vi "_Read_D.vi"(8 "error in (no error)":errorcluster, 11 "Postgres Connector In":refnum<class "Postgres Connector.lvclass">) -> (0 "error out":errorcluster, 3 "Postgres Connector Out":refnum<class "Postgres Connector.lvclass">)   [LabVIEW 2019, in "PG_LIB.lvlib" / "Postgres Connector.lvclass"]
doc: "This VI decode the \"D\" section of the message sent by the database and return the value of each rows."
uses:
  Postgres Connector.lvclass
  Enum_RowDescription_State_Machine.ctl
  Cluster_Reader_Infos.ctl
  Postgres Connector.lvclass/Postgres Connector.ctl
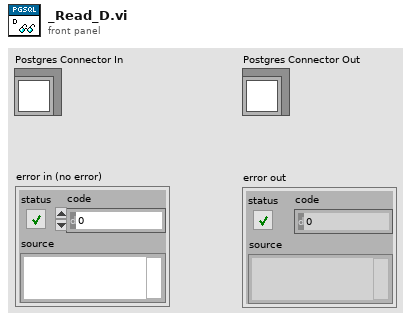
[diagram p1: front panel]
types:
  T1 = typedef "PG_LIB.lvlib/Postgres Connector.lvclass/Cluster_Reader_Infos.ctl" = cluster{"Byte Length":i32}
  T2 = typedef "PG_LIB.lvlib/Postgres Connector.lvclass/Enum_RowDescription_State_Machine.ctl" = enum16{"Check For Error", "Wait For T", "Wait For D", "Wait For Z", "C Byte Length", "Z Byte Length", "n Byte Length", "Byte Length", "Get Infos", "Check For End", "Flush", "Quit"}
  T3 = enum16{"Standard", "Buffered", "CRLF", "Immediate"}
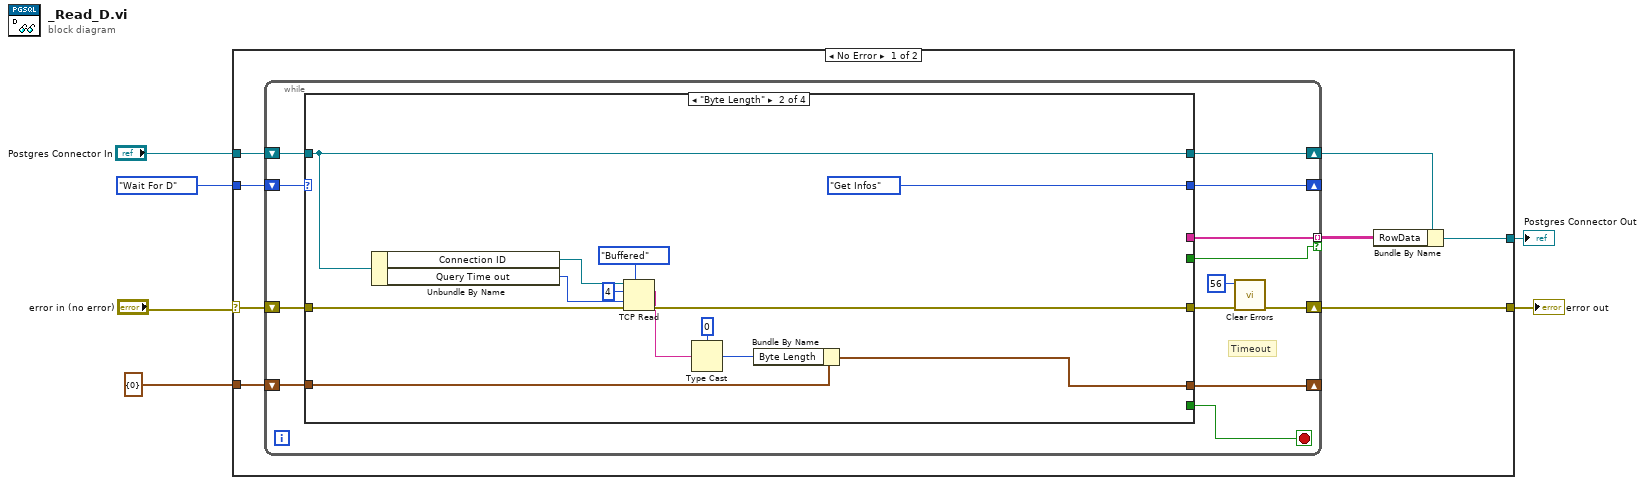
[diagram p0: block diagram]
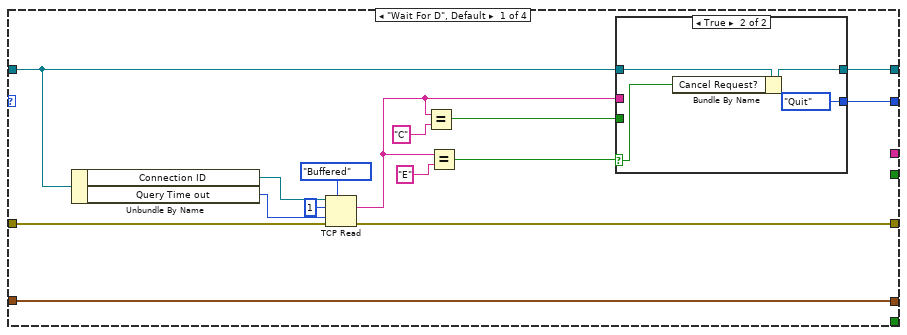
[diagram p2: hidden frame]
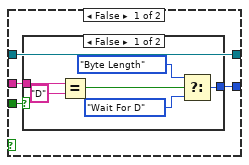
[diagram p3: hidden frame]
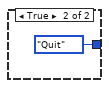
[diagram p4: hidden frame]
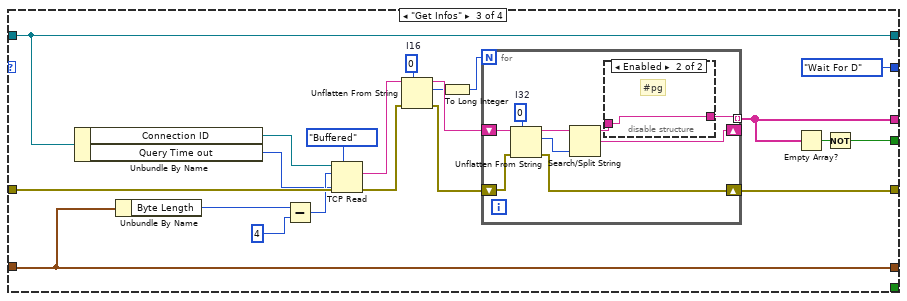
[diagram p5: hidden frame]
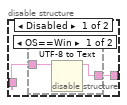
[diagram p6: hidden frame]
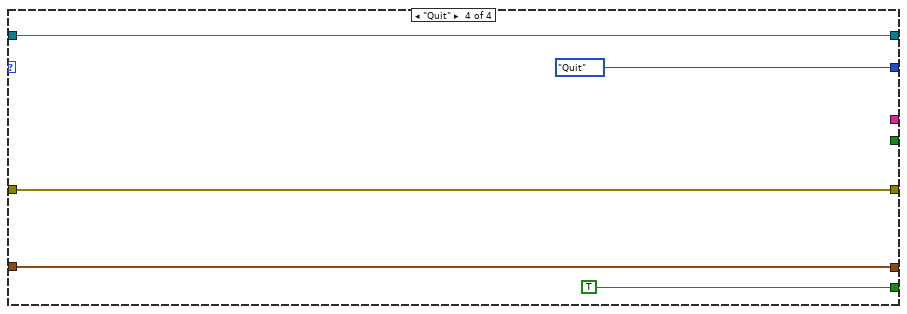
[diagram p8: hidden frame]
diagram:
  n1 = case shown="No Error" "error in (no error)" {
    selector: "error in (no error)" -> [w14 w113]
    tunnel: "Postgres Connector In" -> [w10 w112]
    tunnel: Enum_RowDescription_State_Machine."Wait For D" -> [w13 _]
    tunnel: [w12 w113] -> w3
    tunnel: T1 {"Byte Length"=0} ("Reader_Infos") -> [w11 _]
    tunnel: [w8 w112] -> w1
    frame No Error {
      n2 = while {
        shift-right: [w23] -> w12
        shift-left: w14 -> [w26]
        shift-right: [w21] -> _
        shift-left: w13 -> [w25]
        shift-right: [w19] -> _
        shift-left: w11 -> [w20]
        tunnel: [w17] -> w9 mode=indexing if=w16
        shift-right: [w15] -> w7
        shift-left: w10 -> [w27]
        stop <- w18 stop-if-true
        # "Timeout"
        n3 = case shown="\"Byte Length\"" w25 {
          tunnel: w27 -> [w29 w67 w83 w107]
          tunnel: w26 -> [w39 w66 w89 w110]
          tunnel: [w38 w65 w73 w110] -> w24
          tunnel: [w37 Enum_RowDescription_State_Machine."Get Infos" Enum_RowDescription_State_Machine."Wait For D" Enum_RowDescription_State_Machine."Quit"] -> w21
          tunnel: w20 -> [w36 w63 w87 w111]
          tunnel: [w36 w62 w87 w111] -> w19
          tunnel: [_ _ _ TRUE] -> w18
          tunnel: [_ _ w77 _] -> w17
          tunnel: [_ _ w81 _] -> w16
          tunnel: [w28 w67 w83 w107] -> w15
          frame "Wait For D", Default {
            n4 = Unbundle By Name(w29) -> ("Connection ID"=w41:refnum<k5>, "Query Time out"=w33:i32)
            n5 = TCP Read(connection ID=w41, bytes to read=1, error in (no error)=w39, 7:T3."Buffered" ("mode (standard)"), 9:w33) -> (data out=w31:string, error out=w38:errorcluster)  [unwired: 1 out]
            n6 = Equal?(x=w31, y="C") -> (x = y?=w34:bool)
            n7 = Equal?(x=w31, y="E") -> (x = y?=w30:bool)
            n8 = case shown="True" w30 {
              selector: w30 -> [_ w55]
              tunnel: [w46 Enum_RowDescription_State_Machine."Quit"] -> w37
              tunnel: w34 -> [w45 _]
              tunnel: w31 -> [w44 _]
              tunnel: w29 -> [w43 w56]
              tunnel: [w43 w54] -> w28
              frame False {
                n9 = case shown="False" w45 {
                  tunnel: [w50 Enum_RowDescription_State_Machine."Quit"] -> w46
                  tunnel: w44 -> [w47 _]
                  frame False {
                    n10 = Equal?(x=w47, y="D") -> (x = y?=w51:bool)
                    n11 = Select(t=Enum_RowDescription_State_Machine."Byte Length", s=w51, f=Enum_RowDescription_State_Machine."Wait For D") -> (s? t:f=w50:T2)
                  }
                  frame True {
                  }
                }
              }
              frame True {
                n12 = Bundle By Name(cluster=w56, "Cancel Request?"=w55) -> (w54:refnum<class "Postgres Connector.lvclass">)
              }
            }
          }
          frame "Byte Length" {
            n13 = Unbundle By Name(w67) -> ("Connection ID"=w69:refnum<k5>, "Query Time out"=w58:i32)
            n14 = TCP Read(connection ID=w69, bytes to read=4, error in (no error)=w66, 7:T3."Buffered" ("mode (standard)"), 9:w58) -> (data out=w60:string, error out=w65:errorcluster)  [unwired: 1 out]
            n15 = Type Cast(type=0, x=w60) -> (*(type *) &x=w59:i32)
            n16 = Bundle By Name(cluster=w63, "Byte Length"=w59) -> (w62:T1)
          }
          frame "Get Infos" {
            w80 = i16 0  # I16
            n17 = Unbundle By Name(w83) -> ("Connection ID"=w90:refnum<k5>, "Query Time out"=w74:i32)
            n18 = Unbundle By Name(w87) -> ("Byte Length"=w86:i32)
            n19 = Subtract(x=w86, y=4 ("bytes to read")) -> (x-y=w85:i32)
            n20 = TCP Read(connection ID=w90, bytes to read=w85, error in (no error)=w89, 7:T3."Buffered" ("mode (standard)"), 9:w74) -> (data out=w79:string, error out=w72:errorcluster)  [unwired: 1 out]
            n21 = Unflatten From String(type=w80, binary string=w79, error in (no error)=w72) -> (rest of the binary string=w78:string, value=w76:i16, error out=w71:errorcluster)  [unwired: 2 in]
            n22 = To Long Integer(number=w76) -> (32bit integer=w75:i32)
            n23 = for {
              N: w75 -> [_]
              tunnel: [w92] -> w77 mode=indexing
              shift-right: [w96] -> _
              shift-left: w78 -> [w99]
              shift-right: [w94] -> w73
              shift-left: w71 -> [w95]
              w100 = 0  # I32
              n24 = Unflatten From String(type=w100, binary string=w99, error in (no error)=w95) -> (rest of the binary string=w97:string, value=w98:i32, error out=w94:errorcluster)  [unwired: 2 in]
              n25 = Search/Split String(string=w97, offset (0)=w98) -> (substring before match=w93:string, match + rest of string=w96:string)  [unwired: 1 in, 1 out]
              n26 = disable-structure shown="Enabled" {
                disable-tunnel: w93 -> [w102 w106]
                disable-tunnel: [w101 w106] -> w92
                frame Disabled {
                  n27 = disable-structure shown="OS==Win" {
                    disable-tunnel: w102 -> [w104 w105]
                    disable-tunnel: [w103 w105] -> w101
                    frame condition #0 {
                      n28 = UTF-8 to Text(11:w104) -> (3:w103:string)  [unwired: 2 in, 1 out]
                    }
                    frame condition #1 (active) {
                    }
                  }
                }
                frame Enabled {
                  # "#pg"
                }
              }
            }
            n29 = Empty Array?(array=w77) -> (empty?=w82:bool)
            n30 = Not(x=w82) -> (.not. x?=w81:bool)
          }
          frame "Quit" {
          }
        }
        n31 = call <vilib>:"Clear Errors.vi"("error in (no error)"=w24, "specific error code to clear (0: all)"=56) -> ("error out"=w23:errorcluster)  [unwired: 4 in, 1 out]
      }
      n32 = Bundle By Name(cluster=w7, "RowData"=w9) -> (w8:refnum<class "Postgres Connector.lvclass">)
    }
    frame Error {
    }
  }
  "error out" <- w3
  "Postgres Connector Out" <- w1
